vi "Drive Path Calibrations.vi"() -> ()   [LabVIEW 2016]
panel:
  out "Right Drive Path Derivative Gain":dbl
  out "Right Drive Path Feed-Forward Gain":dbl=0.42
  out "Right Drive Path Proportional Gain":dbl=0.6
  out "Right Drive Path Integral Gain":dbl
  out "Left Drive Path Derivative Gain":dbl
  out "Left Drive Path Feed-Forward Gain":dbl=0.42
  in  "Drive Path Calibrations File Location":path=path "C:/ni-rt/startup/DrivePathCalibrations.txt"
  out "Left Drive Path Proportional Gain":dbl=0.6
  out "Left Drive Path Integral Gain":dbl
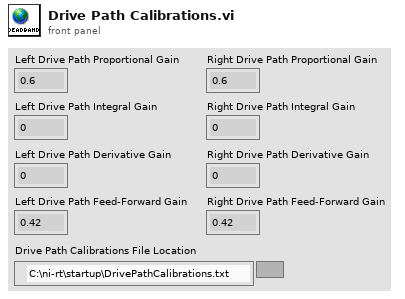
[diagram p1: front panel]
diagram:
